vi "MH_GetErrorString.vi"(8 "error in (no error)":errorcluster, 10 "code":i32) -> (0 "error out":errorcluster, 2 "Error":string, 3 "return type":i32)   [LabVIEW 2019]
uses:
  <userlib>/MultiHarp150/MH_DllPath_global.vi
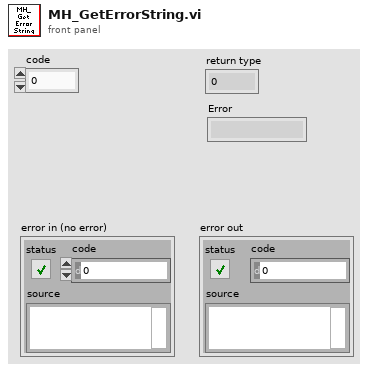
[diagram p1: front panel]
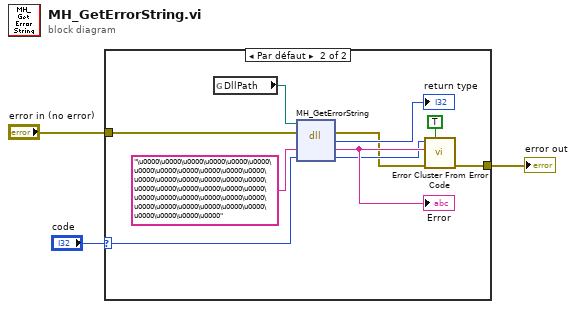
[diagram p0: block diagram]
diagram:
  n1 = case shown="Par défaut" "code" {
    selector: "code" -> [_ w7]
    tunnel: [w4 w8] -> w3
    tunnel: "error in (no error)" -> [w4 w6]
    frame 0 {
    }
    frame Default {
      n2 = global read "MH_DllPath_global.vi" "DllPath"() -> (w14:path)
      n3 = dll-call lib="MHLib64.dll" fn="MH_GetErrorString"(path in=w14, error in=w6, "Error"="\u0000\u0000\u0000\u0000\u0000\u0000\u0000\u0000\u0000\u0000\u0000\u0000\u0000\u0000\u0000\u0000\u0000\u0000\u0000\u0000\u0000\u0000\u0000\u0000\u0000\u0000\u0000\u0000\u0000\u0000\u0000\u0000\u0000\u0000\u0000\u0000\u0000\u0000\u0000\u0000" ("Version"), "code"=w7) -> (error out=w9:errorcluster, "return type"=→"return type":i32, "Error"=w11:string, "code"=w10:i32)  [unwired: 1 in, 1 out]
      "Error" <- w11
      n4 = call <vilib>:"Error Cluster From Error Code.vi"("show call chain? (False)"=TRUE, "error in (no error)"=w9, "error message (\"\")"=w11, "error code (0)"=w10) -> ("error out"=w8:errorcluster)  [unwired: 5 in]
    }
  }
  "error out" <- w3
